vi "SENS_IF_FILT_SAMP_COUN_MODE.vi"(0 "VISA IN":refnum<visa-resource-name>, 1 "AUTO or MANUAL":string(combo)="AUTO", 5 "error in":errorcluster, 7 "Channel":i32) -> (14 "VISA Out":refnum<visa-resource-name>, 19 "error out":errorcluster)   [LabVIEW 2018, in "PNA-X.lvlib"]
uses:
  PNA-X.lvlib
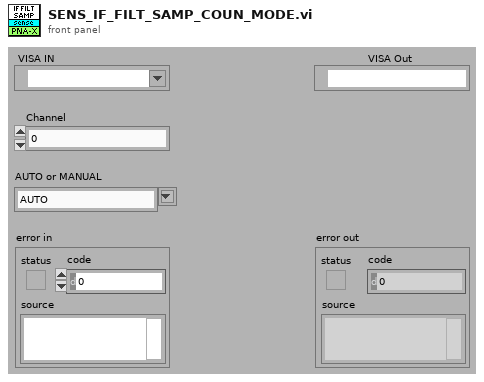
[diagram p1: front panel]
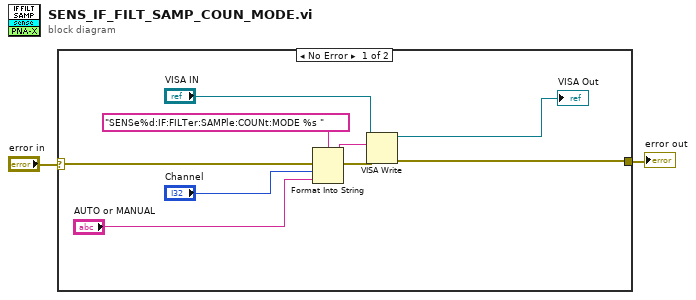
[diagram p0: block diagram]
diagram:
  n1 = case shown="No Error" "error in" {
    selector: "error in" -> [w11 w12]
    tunnel: [w5 w12] -> w1
    frame No Error {
      n2 = Format Into String(format string="SENSe%d:IF:FILTer:SAMPle:COUNt:MODE %s " ("Cmdline"), error in=w11, "Channel", "AUTO or MANUAL") -> (resulting string=w9:string, error out=w10:errorcluster)  [unwired: 1 in]
      n3 = VISA Write(VISA resource name="VISA IN", write buffer=w9, error in (no error)=w10) -> (VISA resource name out=→"VISA Out":refnum<visa-resource-name>, error out=w5:errorcluster)  [unwired: 1 out]
    }
    frame Error {
    }
  }
  "error out" <- w1
